vi "BLAS2 Utility.vi"   [LabVIEW 2020, in "NI_AALBLAS.lvlib"]
uses:
  <vilib>/Analysis/NI_AALBLAS.lvlib
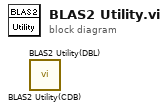
[diagram p0: block diagram]
diagram:
  n1 = call <vilib>:"BLAS2 Utility(CDB).vi"() -> ()  [unwired: 17 in, 3 out]
  n2 = call <vilib>:"BLAS2 Utility(DBL).vi"() -> ()  [unwired: 17 in, 3 out]
